vi "Dump Arrival Time Buffer TIO.vi"(8 "error in":errorcluster, 9 "Number of Photons Counted":i32, 10 "Buffer In":i32[][](array[numeric]), 11 "Temp File Definition":T1) -> (0 "error out":errorcluster, 1 "Number of Photons Counted Out":i32, 3 "Temp File Definition Out":T1)   [LabVIEW 2009]
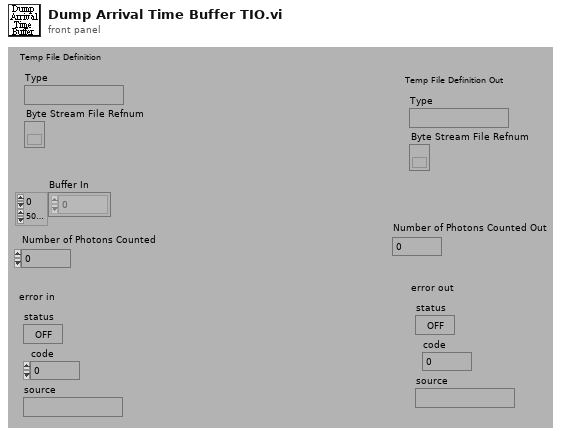
[diagram p1: front panel]
types:
  T1 = cluster{"Type":string, "Byte Stream File Refnum":refnum<file>}
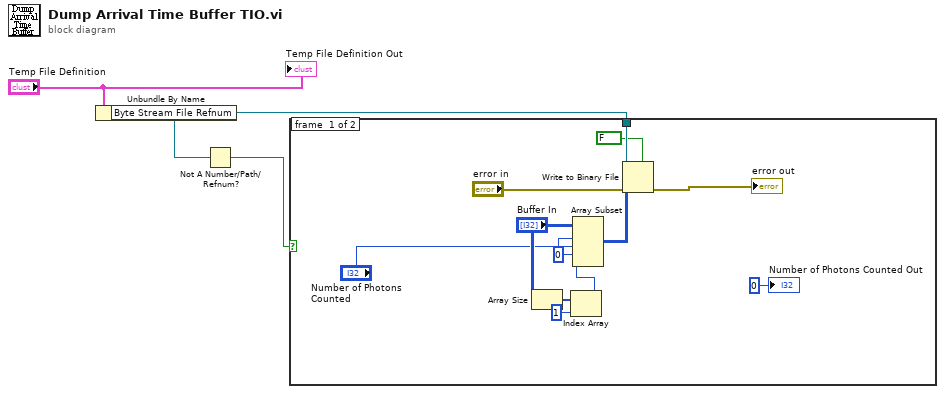
[diagram p0: block diagram]
diagram:
  n1 = Unbundle By Name("Temp File Definition") -> ("Byte Stream File Refnum"=w2:refnum<file>)
  n2 = Not A Number/Path/Refnum?(number/path/refnum=w2) -> (NaN/Path/Refnum?=w1:bool)
  n3 = case shown="False" w1 {
    tunnel: w2 -> [w5 _]
    frame #0 {
      w12 = 0 ("Array Index")
      n4 = Array Size(array="Buffer In") -> (size(s)=w10:i32[])
      n5 = Index Array(array=w10, index=1 ("Index")) -> (element=w8:i32)
      n6 = Array Subset(array="Buffer In", index (row)=w12, length (row)="Number of Photons Counted", index (col)=w12, length (col)=w8) -> (w15:i32[][])
      n7 = Write to Binary File(file (use dialog)=w5, data=w15, error in="error in", 5:FALSE ("prepend array or string size? (T)")) -> (error out=→"error out":errorcluster)  [unwired: 2 in, 2 out]
      "Number of Photons Counted Out" <- 0 ("Number of Photons Counted Out")
    }
    frame #1 {
    }
  }
  "Temp File Definition Out" <- "Temp File Definition"
